vi "DAQ_Digital Pulse Gen Close.vi"(0 "DAQmx Task In":refnum<k21>, 11 "error in":errorcluster) -> (15 "error out":errorcluster)   [LabVIEW 2021, in "DAQ_Digital Pulse Generation.lvlib"]
doc: "Aborts and clears the Digital Pulse Generation task"
uses:
  DAQ_Digital Pulse Generation.lvlib
panel:
  # "Inputs"
  # "Outputs"
  # "Overview:\nThis VI closes the digitial pulse generation DAQmx Task.\n\nHardware Requirement: A compatible PXI, PCIe, USB, cDAQ or Testscale device\n\nSoftware Requirement: NI DAQmx 2022Q4 or later\n\n\nInstructions:\n1. Input the digitial pulse generation task through DAQmx Task In control.\n2. This VI aborts and clears the digitial pulse generation task."
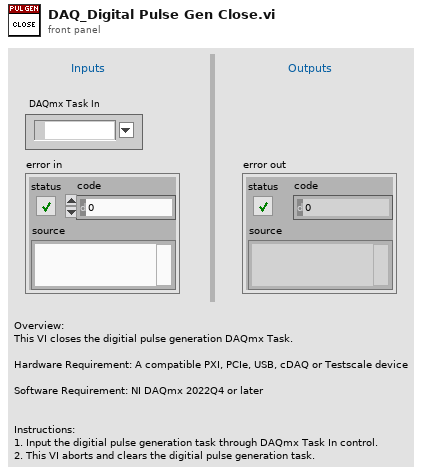
[diagram p1: front panel]
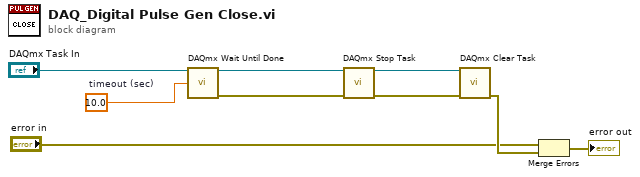
[diagram p0: block diagram]
diagram:
  w1 = 10.0  # timeout (sec)
  n1 = call <vilib>:"DAQmx Wait Until Done.vi"("task/channels in"="DAQmx Task In", "timeout (sec)"=w1) -> ("task out"=w3:refnum<k21>, "error out"=w2:errorcluster)  [unwired: 12 in]
  n2 = call <vilib>:"DAQmx Stop Task.vi"("task/channels in"=w3, "error in"=w2) -> ("task out"=w8:refnum<k21>, "error out"=w7:errorcluster)  [unwired: 12 in]
  n3 = call <vilib>:"DAQmx Clear Task.vi"("task in"=w8, "error in"=w7) -> ("error out"=w5:errorcluster)  [unwired: 13 in]
  n4 = Merge Errors("error in", w5) -> (→"error out":errorcluster)
